vi "Properties_Insert Dividers.vi"(11 "Property Info Array In":T1(array[cluster])) -> (2 "Divider Ct":i32, 3 "Property Info Array Out":T1(array[cluster]))   [LabVIEW 2023]
doc: "Insert Divider Element between each major class type. This is used for display and also for reversing the class order in the BundleMagoc dialog.\n\nThis must come before dotted properties are inserted."
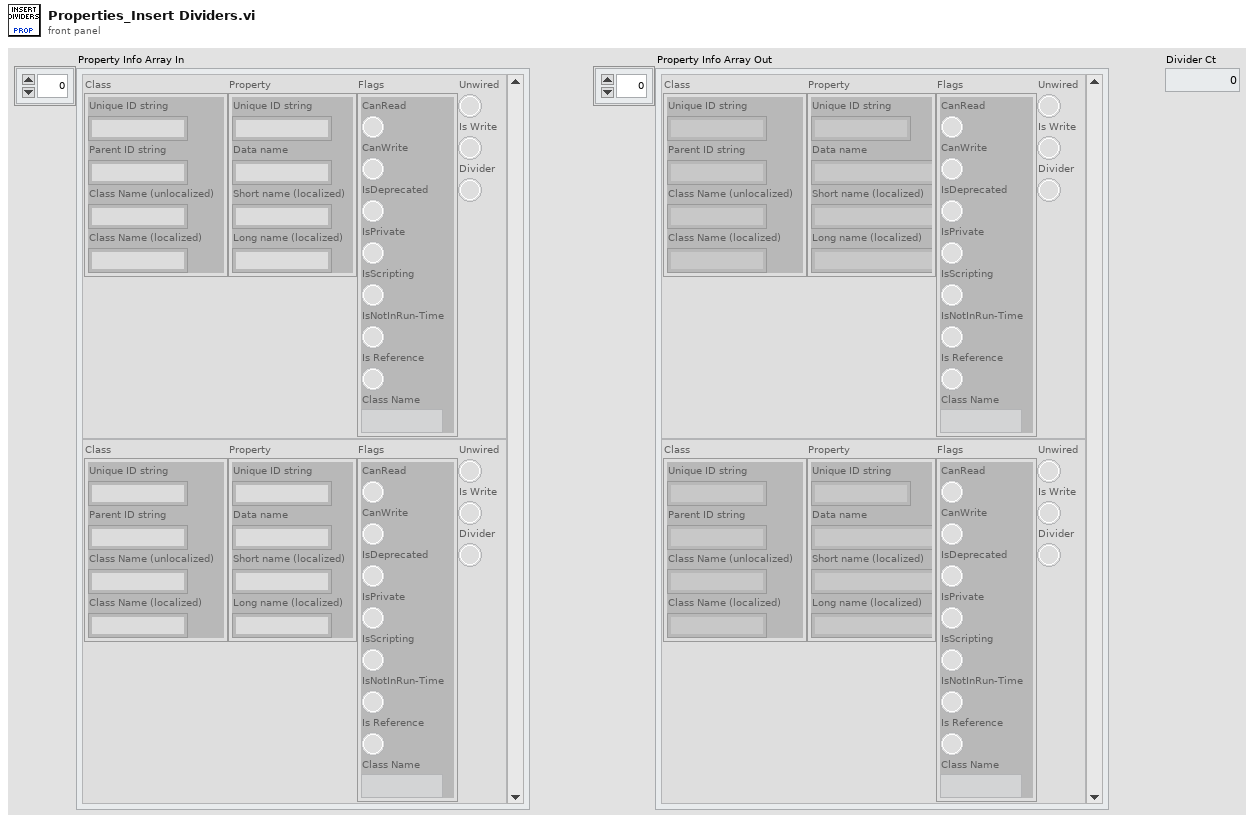
[diagram p1: front panel]
types:
  T1 = cluster{"Class":cluster{"Unique ID string":string, "Parent ID string":string, "Class Name (unlocalized)":string, "Class Name (localized)":string}, "Property":cluster{"Unique ID string":string, "Data name":string, "Short name (localized)":string, "Long name (localized)":string}, "Flags":cluster{"CanRead":bool, "CanWrite":bool, "IsDeprecated":bool, "IsPrivate":bool, "IsScripting":bool, "IsNotInRun-Time":bool, "Is Reference":bool, "Class Name":string}, "Divider":bool, "Is Write":bool, "Unwired":bool}[]
  T2 = cluster{"Class":cluster{"Unique ID string":string, "Parent ID string":string, "Class Name (unlocalized)":string, "Class Name (localized)":string}, "Property":cluster{"Unique ID string":string, "Data name":string, "Short name (localized)":string, "Long name (localized)":string}, "Flags":cluster{"CanRead":bool, "CanWrite":bool, "IsDeprecated":bool, "IsPrivate":bool, "IsScripting":bool, "IsNotInRun-Time":bool, "Is Reference":bool, "Class Name":string}, "Divider":bool, "Is Write":bool, "Unwired":bool}
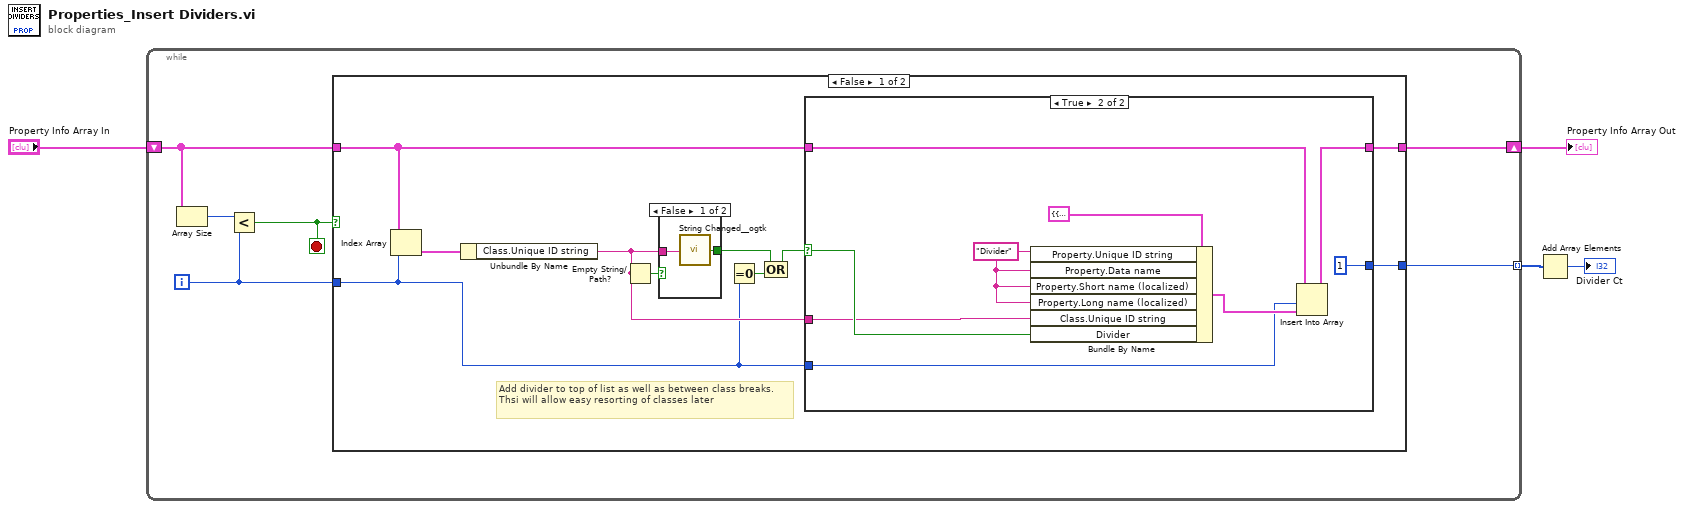
[diagram p0: block diagram]
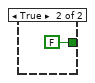
[diagram p2: hidden frame]
diagram:
  n1 = while {
    shift-right: [w6] -> w3
    shift-left: "Property Info Array In" -> [w10]
    tunnel: [w7] -> w2 mode=indexing
    i -> [w8]
    stop <- w5 stop-if-true
    n2 = Array Size(array=w10) -> (size(s)=w9:i32)
    n3 = Less?(x=w9, y=w8) -> (x < y?=w5:bool)
    n4 = case shown="False" w5 {
      tunnel: [w20 w34] -> w6
      tunnel: w10 -> [w19 w34]
      tunnel: w8 -> [w14 _]
      tunnel: [w18 _] -> w7
      frame False {
        # "Add divider to top of list as well as between class breaks. Thsi will allow easy resorting of classes later"
        n5 = Index Array(array=w19, index=w14) -> (element=w16:T2)
        n6 = Unbundle By Name(w16) -> ("Class.Unique ID string"=w15:string)
        n7 = Empty String/Path?(string/path=w15) -> (empty?=w17:bool)
        n8 = case shown="False" w17 {
          tunnel: w15 -> [w22 _]
          tunnel: [w21 FALSE ("Changed")] -> w12
          frame False {
            n9 = call <userlib>:"String Changed__ogtk.vi"("String"=w22) -> ("Changed"=w21:bool)
          }
          frame True {
          }
        }
        n10 = Equal To 0?(x=w14) -> (x = 0?=w13:bool)
        n11 = Compound Arithmetic op=OR(w12, w13) -> (w11:bool)
        n12 = case shown="True" w11 {
          selector: w11 -> [_ w29]
          tunnel: [w24 w33] -> w20
          tunnel: w19 -> [w24 w32]
          tunnel: w14 -> [_ w27]
          tunnel: [_ 1] -> w18
          tunnel: w15 -> [_ w26]
          frame False {
          }
          frame True {
            w25 = "Divider" ("Property.Unique ID string")
            n13 = Bundle By Name(cluster=T2 {"Class"={"Unique ID string"="", "Parent ID string"="", "Class Name (unlocalized)"="", "Class Name (localized)"=""}, "Property"={"Unique ID string"="", "Data name"="", "Short name (localized)"="", "Long name (localized)"=""}, "Flags"={"CanRead"=FALSE, "CanWrite"=FALSE, "IsDeprecated"=FALSE, "IsPrivate"=FALSE, "IsScripting"=FALSE, "IsNotInRun-Time"=FALSE, "Is Reference"=FALSE, "Class Name"=""}, "Divider"=FALSE, "Is Write"=FALSE, "Unwired"=FALSE}, "Property.Unique ID string"=w25, "Property.Data name"=w25, "Property.Short name (localized)"=w25, "Property.Long name (localized)"=w25, "Class.Unique ID string"=w26, "Divider"=w29) -> (w28:T2)
            n14 = Insert Into Array(array=w32, index=w27, new element=w28) -> (w33:T1)
          }
        }
      }
      frame True {
      }
    }
  }
  "Property Info Array Out" <- w3
  n15 = Add Array Elements(numeric array=w2) -> (sum=→"Divider Ct":i32)
